vi "Get Limit Value Numeric.vi"(8 "error in (no error)":errorcluster, 9 "Limit":enum16{"LIMIT1", "LIMIT2"}(ring), 10 "Step Output in":T1, 11 "Execution in":refnum<data-value>) -> (0 "error out":errorcluster, 2 "Limit Value":dbl, 3 "Execution out":refnum<data-value>)   [LabVIEW 2015, in "Execution.lvclass"]
uses:
  Execution.lvclass
  Step/STEP_OUTPUT.ctl
  Step/OUTPUT_DATA_TYPE.ctl
  OutputUI/OUTPUT_CHECK_TYPE.ctl
  Step/OUTPUT_VALUE_TYPE.ctl
  <vilib>/Utility/Data Type/NI_Data Type.lvlib
  Step.lvclass
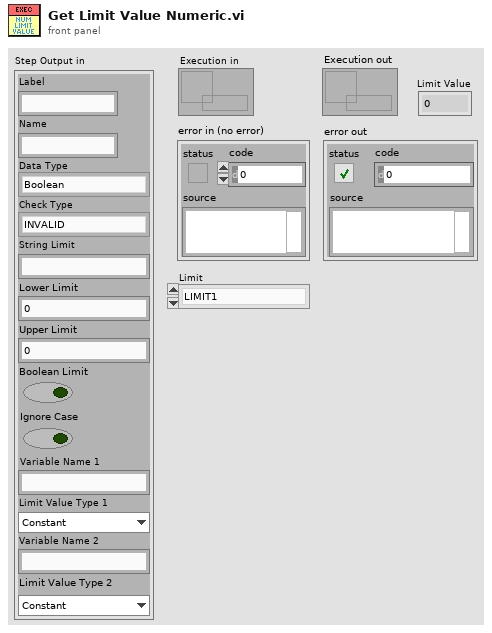
[diagram p1: front panel]
types:
  T1 = typedef "Step.lvclass/STEP_OUTPUT.ctl" = cluster{"Label":string, "Name":string, "Data Type":T2, "Check Type":T3, "String Limit":string, "Lower Limit":dbl, "Upper Limit":dbl, "Boolean Limit":bool, "Ignore Case":bool, "Variable Name 1":string, "Limit Value Type 1":T4, "Variable Name 2":string, "Limit Value Type 2":T4}
  T2 = typedef "Step.lvclass/OUTPUT_DATA_TYPE.ctl" = enum16{"Boolean", "String", "Numeric", "Other"}
  T3 = typedef "Step.lvclass/OUTPUT_CHECK_TYPE.ctl" = enum16{"INVALID", "DO_NOT_CHECK", "RECORD", "VARIABLE", "EQUAL", "NOT_EQUAL", "STR_CONTAINS", "STR_START_WITH", "STR_END_WITH", "STR_REGEX_MATCH", "NUM_GT", "NUM_LT", "NUM_GE", "NUM_LE", "NUM_RANGE", "NUM_RANGE_BDY"}
  T4 = typedef "Step.lvclass/OUTPUT_VALUE_TYPE.ctl" = enum16{"Constant", "Variable"}
  T5 = typedef "NI_Data Type.lvlib/Data Type.ctl" = enum8{"Invalid Type", "Void", "I8", "I16", "I32", "I64", "U8", "U16", "U32", "U64", "Single Float", "Double Float", "Extended Float", "Single Complex", "Double Complex", "Extended Complex", "Enum U8", "Enum U16", "Enum U32", "Enum U64", "Single Float With Unit", "Double Float With Unit", "Extended Float With Unit", "Single Complex with Unit", "Double Complex with Unit", "Extended Complex with Unit", "Boolean", "String", "Path", "Picture", "Tag", "Array", "Cluster", "Variant", "LV Variant", "Waveform", "Timestamp", "Digital Waveform", "Digital Data", "ExpressData", "Refnum", "External Data", "VI", "Poly VI", "LabVIEW Class Instance", "Fixed Point"}
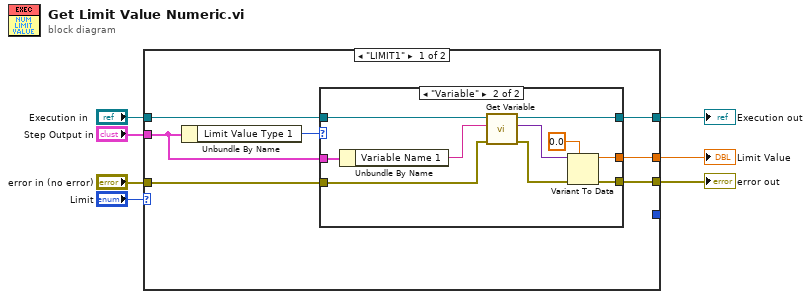
[diagram p0: block diagram]
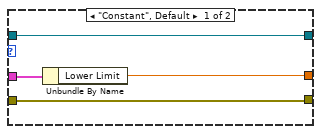
[diagram p2: hidden frame]
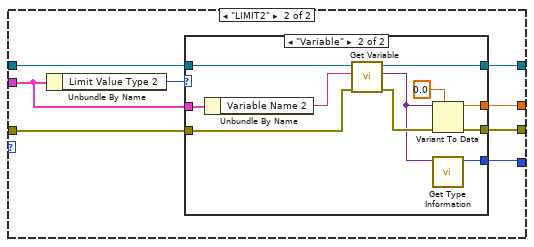
[diagram p3: hidden frame]
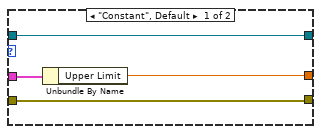
[diagram p4: hidden frame]
diagram:
  n1 = case shown="\"LIMIT1\"" "Limit" {
    tunnel: "Step Output in" -> [w14 w36]
    tunnel: "Execution in" -> [w12 w34]
    tunnel: [w11 w33] -> w5
    tunnel: [w10 w32] -> w4
    tunnel: [w9 w31] -> w3
    tunnel: "error in (no error)" -> [w8 w30]
    tunnel: [_ w29] -> _
    frame "LIMIT1" {
      n2 = Unbundle By Name(w14) -> ("Limit Value Type 1"=w13:T4)
      n3 = case shown="\"Variable\"" w13 {
        tunnel: w12 -> [w17 w28]
        tunnel: [w17 w27] -> w11
        tunnel: w14 -> [w18 w21]
        tunnel: [w16 w23] -> w10
        tunnel: [w15 w22] -> w9
        tunnel: w8 -> [w15 w19]
        frame "Constant", Default {
          n4 = Unbundle By Name(w18) -> ("Lower Limit"=w16:dbl)
        }
        frame "Variable" {
          n5 = Unbundle By Name(w21) -> ("Variable Name 1"=w20:string)
          n6 = call "Get Variable.vi"("error in (no error)"=w19, "Name"=w20, "Execution in"=w28) -> ("error out"=w26:errorcluster, "Value"=w25:variant, "Execution out"=w27:refnum<data-value>)  [unwired: 6 in]
          n7 = Variant To Data(error in=w26, type=0.0, Variant=w25) -> (data=w23:dbl, error out=w22:errorcluster)
        }
      }
    }
    frame "LIMIT2" {
      n8 = Unbundle By Name(w36) -> ("Limit Value Type 2"=w35:T4)
      n9 = case shown="\"Variable\"" w35 {
        tunnel: w34 -> [w39 w51]
        tunnel: [w39 w50] -> w33
        tunnel: w36 -> [w40 w45]
        tunnel: [w38 w47] -> w32
        tunnel: [w37 w46] -> w31
        tunnel: w30 -> [w37 w43]
        tunnel: [_ w41] -> w29
        frame "Constant", Default {
          n10 = Unbundle By Name(w40) -> ("Upper Limit"=w38:dbl)
        }
        frame "Variable" {
          n11 = Unbundle By Name(w45) -> ("Variable Name 2"=w44:string)
          n12 = call "Get Variable.vi"("error in (no error)"=w43, "Name"=w44, "Execution in"=w51) -> ("error out"=w49:errorcluster, "Value"=w42:variant, "Execution out"=w50:refnum<data-value>)  [unwired: 6 in]
          n13 = Variant To Data(error in=w49, type=0.0, Variant=w42) -> (data=w47:dbl, error out=w46:errorcluster)
          n14 = call <vilib>:"Get Type Information.vi"("Variant"=w42) -> ("Type"=w41:T5)  [unwired: 6 in, 4 out]
        }
      }
    }
  }
  "Execution out" <- w5
  "Limit Value" <- w4
  "error out" <- w3
